vi "Get Fit Settings.vi"(6 "Fit Model":T2, 8 "Error In":errorcluster, 9 "Additional Parameters":variant, 10 "Fixed Parameters":T1, 11 "XY Graph Ref":refnum<vi>) -> (0 "Error Out":errorcluster, 2 "Additional Fit Settings":variant, 3 "LM Function & Gradient":refnum<vi>)   [LabVIEW 2019]
uses:
  Fit Models.ctl
  D-Only Fixed Parameters.ctl
  N Components Additional Fit Settings.ctl
  Variant/Variant to Data/Variant to Data.lvlib
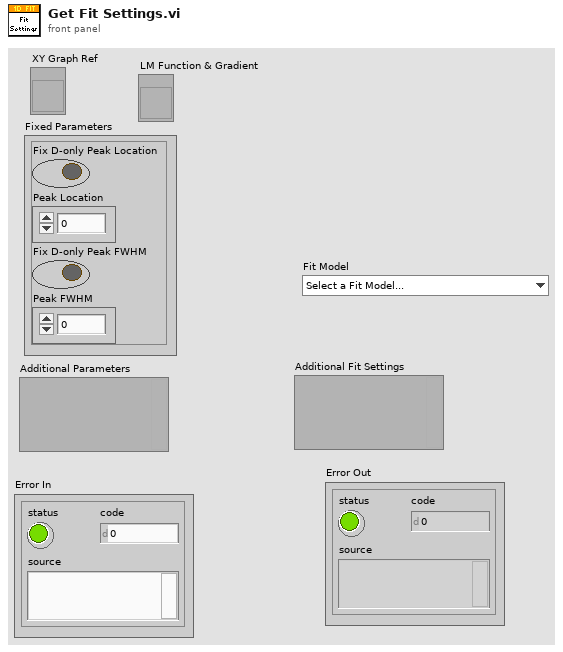
[diagram p1: front panel]
types:
  T1 = typedef "D-Only Fixed Parameters.ctl" = cluster{"Fix D-only Peak Location":bool, "Peak Location":dbl, "Fix D-only Peak FWHM":bool, "Peak FWHM":dbl}
  T2 = typedef "Fit Models.ctl" = enum16{"Select a Fit Model...", "           Single Peak", "Gaussian", "Asymmetric Gaussian", "Lorentzian", "Asymmetric Lorentzian", "Gaussian/Lorentzian", "Lorentzian/Gaussian", "           Double Peak", "Two Gaussians", "Two Asymmetric Gaussians", "Two H-Connected Gaussians", "Two T-Connected Gaussians", "Two H-Connected Asymmetric Gaussians", "Two T-Connected Asymmetric Gaussians", "           Triple Peak", "Three Gaussians", "Three Asymmetric Gaussians", "              Decays", "1-Exponential", "IRF*PSED", "2-Exponentials", "               ACF", "2D Gaussian ACF", "2D Gaussian + Blinking ACF", "2D Gaussian + Flow ACF", "3D Gaussian ACF", "3D Gaussian + Blinking ACF", "             Multiplot", "2D Gaussian ACF & 2D Gaussian + Flow ACF"}
  T3 = typedef "N Components Additional Fit Settings.ctl" = cluster{"Fixed Parameters":T1, "Cursor Coordinates":dbl[], "Data Split Point":i32}
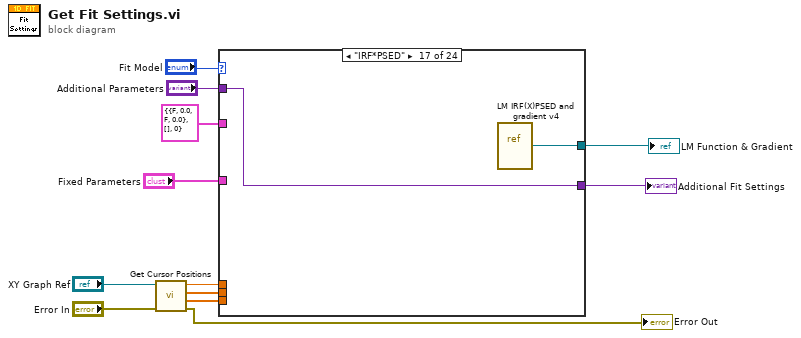
[diagram p0: block diagram]
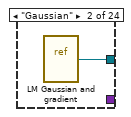
[diagram p3: hidden frame]
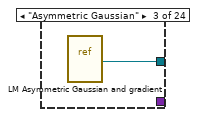
[diagram p4: hidden frame]
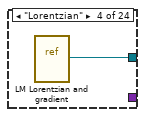
[diagram p5: hidden frame]
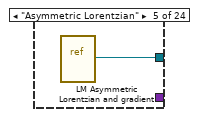
[diagram p6: hidden frame]
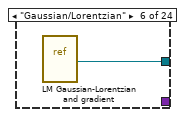
[diagram p7: hidden frame]
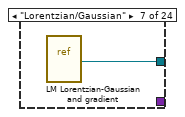
[diagram p8: hidden frame]
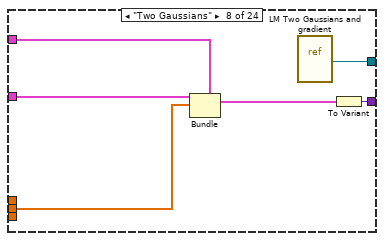
[diagram p9: hidden frame]
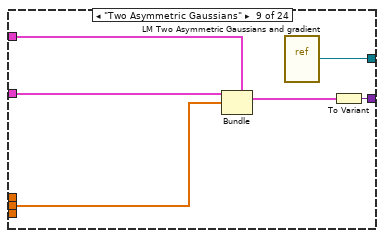
[diagram p10: hidden frame]
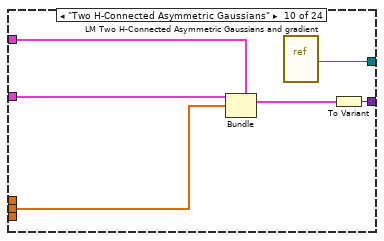
[diagram p11: hidden frame]
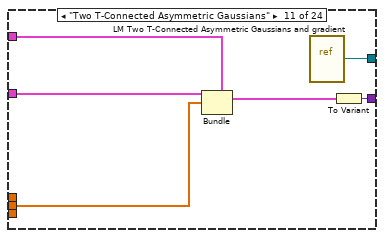
[diagram p12: hidden frame]
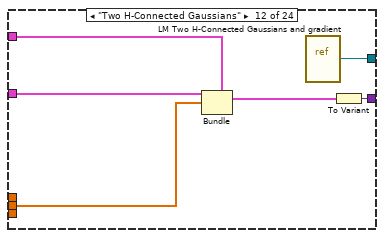
[diagram p13: hidden frame]
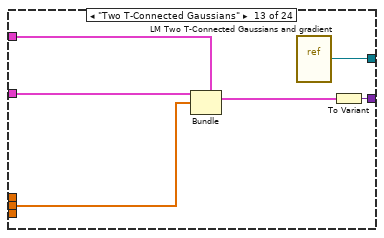
[diagram p14: hidden frame]
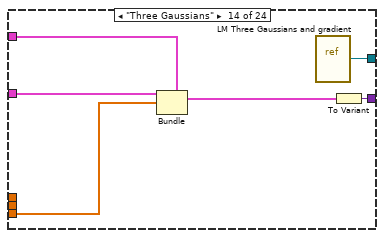
[diagram p15: hidden frame]
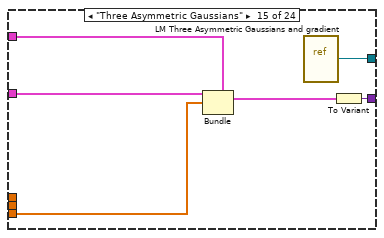
[diagram p16: hidden frame]
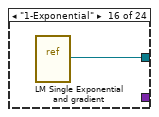
[diagram p17: hidden frame]
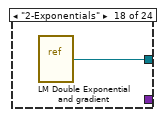
[diagram p18: hidden frame]
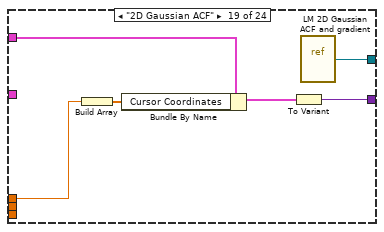
[diagram p19: hidden frame]
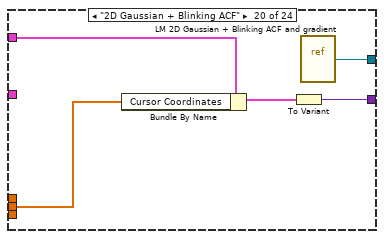
[diagram p20: hidden frame]
diagram:
  n1 = call "Get Cursor Positions.vi"("Error In"="Error In", "XYGraph in"="XY Graph Ref") -> ("Error Out"=→"Error Out":errorcluster, "Cursor 1-3 Positions"=w6:dbl[], "Cursor 1 & 2 Positions"=w7:dbl[], "Cursor 1 Position"=w8:dbl)  [unwired: 6 in]
  n2 = case shown="\"IRF*PSED\"" "Fit Model" {
    tunnel: "Fixed Parameters" -> [_ _ _ _ _ _ _ w24 w30 w36 w42 w48 w54 w60 w66 _ _ _ _ _ _ _ _ _]
    tunnel: [_ _ _ _ _ _ _ w22 w28 w34 w40 w46 w52 w58 w64 _ w68 _ w71 w77 w82 w87 w93 w98] -> w11
    tunnel: w6 -> [_ _ _ _ _ _ _ _ _ _ _ _ _ w57 w63 _ _ _ _ _ _ _ _ _]
    tunnel: w7 -> [_ _ _ _ _ _ _ w21 w27 w33 w39 w45 w51 _ _ _ _ _ _ w80 w85 _ w96 w100]
    tunnel: w8 -> [_ _ _ _ _ _ _ _ _ _ _ _ _ _ _ _ _ _ w76 _ _ w92 _ _]
    tunnel: T3 {"Fixed Parameters"={"Fix D-only Peak Location"=FALSE, "Peak Location"=0.0, "Fix D-only Peak FWHM"=FALSE, "Peak FWHM"=0.0}, "Cursor Coordinates"=[], "Data Split Point"=0} ("N Components Additional Fit Settings") -> [_ _ _ _ _ _ _ w20 w26 w32 w38 w44 w50 w56 w62 _ _ _ w73 w79 w84 w89 w95 w104]
    tunnel: "Additional Parameters" -> [_ _ _ _ _ _ _ _ _ _ _ _ _ _ _ _ w68 _ _ _ _ _ _ w102]
    tunnel: [_ w13 w14 w15 w16 w17 w18 w19 w25 w31 w37 w43 w49 w55 w61 w67 w69 w70 w72 w78 w83 w88 w94 w99] -> w1
    frame "Select a Fit Model...", Default {
    }
    frame "Gaussian" {
      n3 = vi-ref "LM Gaussian and gradient.vi"() -> (w13:refnum<vi>)
    }
    frame "Asymmetric Gaussian" {
      n4 = vi-ref "LM Asymmetric Gaussian and gradient.vi"() -> (w14:refnum<vi>)
    }
    frame "Lorentzian" {
      n5 = vi-ref "LM Lorentzian and gradient.vi"() -> (w15:refnum<vi>)
    }
    frame "Asymmetric Lorentzian" {
      n6 = vi-ref "LM Asymmetric Lorentzian and gradient.vi"() -> (w16:refnum<vi>)
    }
    frame "Gaussian/Lorentzian" {
      n7 = vi-ref "LM Gaussian-Lorentzian and gradient.vi"() -> (w17:refnum<vi>)
    }
    frame "Lorentzian/Gaussian" {
      n8 = vi-ref "LM Lorentzian-Gaussian and gradient.vi"() -> (w18:refnum<vi>)
    }
    frame "Two Gaussians" {
      n9 = Bundle(cluster=w20, "Fixed Parameters"=w24, "Cursor Coordinates"=w21) -> (w23:T3)  [unwired: 1 in]
      n10 = vi-ref "LM Two Gaussians and gradient.vi"() -> (w19:refnum<vi>)
      n11 = To Variant(anything=w23) -> (Variant=w22:variant)
    }
    frame "Two Asymmetric Gaussians" {
      n12 = Bundle(cluster=w26, "Fixed Parameters"=w30, "Cursor Coordinates"=w27) -> (w29:T3)  [unwired: 1 in]
      n13 = vi-ref "LM Two Asymmetric Gaussians and gradient.vi"() -> (w25:refnum<vi>)
      n14 = To Variant(anything=w29) -> (Variant=w28:variant)
    }
    frame "Two H-Connected Asymmetric Gaussians" {
      n15 = Bundle(cluster=w32, "Fixed Parameters"=w36, "Cursor Coordinates"=w33) -> (w35:T3)  [unwired: 1 in]
      n16 = vi-ref "LM Two H-Connected Asymmetric Gaussians and gradient.vi"() -> (w31:refnum<vi>)
      n17 = To Variant(anything=w35) -> (Variant=w34:variant)
    }
    frame "Two T-Connected Asymmetric Gaussians" {
      n18 = Bundle(cluster=w38, "Fixed Parameters"=w42, "Cursor Coordinates"=w39) -> (w41:T3)  [unwired: 1 in]
      n19 = vi-ref "LM Two T-Connected Asymmetric Gaussians and gradient.vi"() -> (w37:refnum<vi>)
      n20 = To Variant(anything=w41) -> (Variant=w40:variant)
    }
    frame "Two H-Connected Gaussians" {
      n21 = Bundle(cluster=w44, "Fixed Parameters"=w48, "Cursor Coordinates"=w45) -> (w47:T3)  [unwired: 1 in]
      n22 = vi-ref "LM Two H-Connected Gaussians and gradient.vi"() -> (w43:refnum<vi>)
      n23 = To Variant(anything=w47) -> (Variant=w46:variant)
    }
    frame "Two T-Connected Gaussians" {
      n24 = Bundle(cluster=w50, "Fixed Parameters"=w54, "Cursor Coordinates"=w51) -> (w53:T3)  [unwired: 1 in]
      n25 = vi-ref "LM Two T-Connected Gaussians and gradient.vi"() -> (w49:refnum<vi>)
      n26 = To Variant(anything=w53) -> (Variant=w52:variant)
    }
    frame "Three Gaussians" {
      n27 = Bundle(cluster=w56, "Fixed Parameters"=w60, "Cursor Coordinates"=w57) -> (w59:T3)  [unwired: 1 in]
      n28 = vi-ref "LM Three Gaussians and gradient.vi"() -> (w55:refnum<vi>)
      n29 = To Variant(anything=w59) -> (Variant=w58:variant)
    }
    frame "Three Asymmetric Gaussians" {
      n30 = Bundle(cluster=w62, "Fixed Parameters"=w66, "Cursor Coordinates"=w63) -> (w65:T3)  [unwired: 1 in]
      n31 = vi-ref "LM Three Asymmetric Gaussians and gradient.vi"() -> (w61:refnum<vi>)
      n32 = To Variant(anything=w65) -> (Variant=w64:variant)
    }
    frame "1-Exponential" {
      n33 = vi-ref "LM Single Exponential and gradient.vi"() -> (w67:refnum<vi>)
    }
    frame "IRF*PSED" {
      n34 = vi-ref "LM IRF(X)PSED and gradient v4.vi"() -> (w69:refnum<vi>)
    }
    frame "2-Exponentials" {
      n35 = vi-ref "LM Double Exponential and gradient.vi"() -> (w70:refnum<vi>)
    }
    frame "2D Gaussian ACF" {
      n36 = Build Array(w76) -> (w75:dbl[])
      n37 = Bundle By Name(cluster=w73, "Cursor Coordinates"=w75) -> (w74:T3)
      n38 = To Variant(anything=w74) -> (Variant=w71:variant)
      n39 = vi-ref "LM 2D Gaussian ACF and gradient.vi"() -> (w72:refnum<vi>)
    }
    frame "2D Gaussian + Blinking ACF" {
      n40 = Bundle By Name(cluster=w79, "Cursor Coordinates"=w80) -> (w81:T3)
      n41 = To Variant(anything=w81) -> (Variant=w77:variant)
      n42 = vi-ref "LM 2D Gaussian + Blinking ACF and gradient.vi"() -> (w78:refnum<vi>)
    }
    frame "2D Gaussian + Flow ACF" {
      n43 = Bundle By Name(cluster=w84, "Cursor Coordinates"=w85) -> (w86:T3)
      n44 = To Variant(anything=w86) -> (Variant=w82:variant)
      n45 = vi-ref "LM 2D Gaussian + Flow ACF and gradient.vi"() -> (w83:refnum<vi>)
    }
    frame "3D Gaussian ACF" {
      n46 = Build Array(w92) -> (w91:dbl[])
      n47 = Bundle By Name(cluster=w89, "Cursor Coordinates"=w91) -> (w90:T3)
      n48 = To Variant(anything=w90) -> (Variant=w87:variant)
      n49 = vi-ref "LM 3D Gaussian ACF and gradient.vi"() -> (w88:refnum<vi>)
    }
    frame "3D Gaussian + Blinking ACF" {
      n50 = Bundle By Name(cluster=w95, "Cursor Coordinates"=w96) -> (w97:T3)
      n51 = To Variant(anything=w97) -> (Variant=w93:variant)
      n52 = vi-ref "LM 3D Gaussian + Blinking ACF and gradient.vi"() -> (w94:refnum<vi>)
    }
    frame "2D Gaussian ACF & 2D Gaussian + Flow ACF" {
      n53 = call "Variant to I32.vi"("Variant"=w102) -> ("Value"=w101:i32)  [unwired: 8 in]
      n54 = Bundle By Name(cluster=w104, "Data Split Point"=w101, "Cursor Coordinates"=w100) -> (w103:T3)
      n55 = vi-ref "LM 2D Gaussian ACF + Flow and gradient (Global).vi"() -> (w99:refnum<vi>)
      n56 = To Variant(anything=w103) -> (Variant=w98:variant)
    }
  }
  "Additional Fit Settings" <- w11
  "LM Function & Gradient" <- w1
